vi "QSM - Invalid.vi"(6 "QSM":T1={"Invalid Option"=enum."Ignore", "QSM"=refnum}, 8 "error in (no error)":errorcluster, 11 "State":string) -> (0 "error out":errorcluster)   [LabVIEW 2014]
doc: "This handles Invalid Cases\n\nDataEtc Copyright (c) 2013"
uses:
  TypeDef/QSM - STYP.ctl
  TypeDef/Invalid Option - STYP.ctl
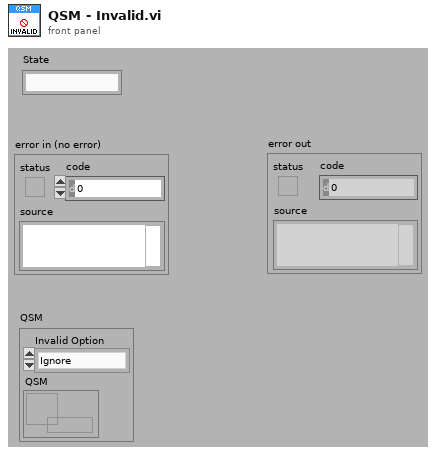
[diagram p1: front panel]
types:
  T1 = typedef "QSM - STYP.ctl" = cluster{"Invalid Option":T2, "QSM":refnum<queue>}
  T2 = typedef "Invalid Option - STYP.ctl" = enum16{"Dialog", "Error", "Ignore"}
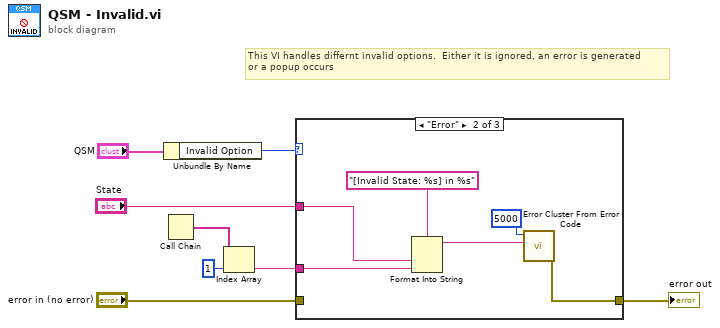
[diagram p0: block diagram]
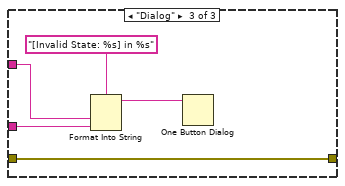
[diagram p3: hidden frame]
diagram:
  # "This VI handles differnt invalid options.  Either it is ignored, an error is generated\nor a popup occurs"
  n1 = Unbundle By Name("QSM") -> ("Invalid Option"=w7:T2)
  n2 = Call Chain() -> (call chain=w6:string[])
  n3 = Index Array(array=w6, index=1) -> (element=w3:string)
  n4 = case shown="\"Error\"" w7 {
    tunnel: "State" -> [_ w14 w19]
    tunnel: w3 -> [_ w13 w18]
    tunnel: "error in (no error)" -> [w9 _ w16]
    tunnel: [w9 w10 w16] -> w1
    frame "Ignore", Default {
    }
    frame "Error" {
      n5 = Format Into String(format string="[Invalid State: %s] in %s", w14, w13) -> (resulting string=w11:string)  [unwired: 2 in, 1 out]
      n6 = call <vilib>:"Error Cluster From Error Code.vi"("error message (\"\")"=w11, "error code (0)"=5000) -> ("error out"=w10:errorcluster)  [unwired: 2 in, 5 out]
    }
    frame "Dialog" {
      n7 = Format Into String(format string="[Invalid State: %s] in %s", w19, w18) -> (resulting string=w17:string)  [unwired: 2 in, 1 out]
      n8 = One Button Dialog(message=w17) -> ()  [unwired: 2 out]
    }
  }
  "error out" <- w1
